vi "Dag 1.vi"() -> ()   [LabVIEW 2015]
panel:
  out "x+y":dbl
  out "Waveform Chart":dbl(graph)
  out "Numeric 2":i32
  out "Boolean 2":bool
  in  "Numeric":dbl
  in  "Boolean":bool
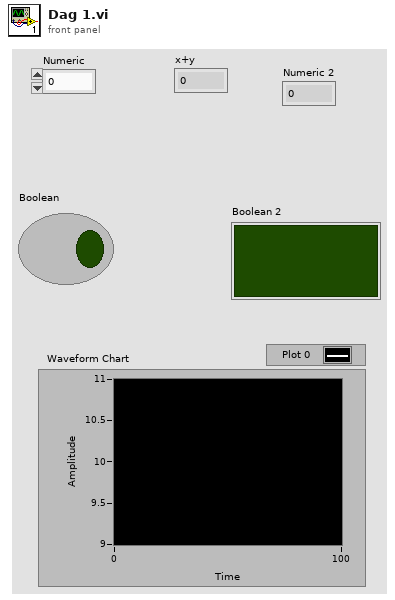
[diagram p1: front panel]
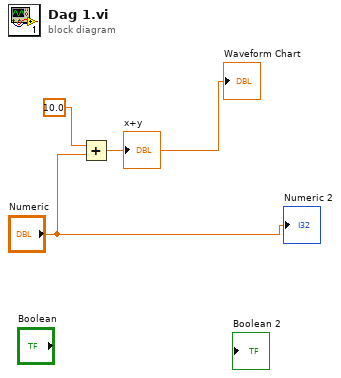
[diagram p0: block diagram]
diagram:
  n1 = Add(x=10.0 ("Numeric"), y="Numeric") -> (x+y=→"Waveform Chart" →"x+y":dbl)
  "Numeric 2" <- "Numeric"
